vi "3D Scan.vi"() -> ()   [LabVIEW 2011]
uses:
  Global 1.vi
panel:
  in  "Path":path
  in  "Save?":bool
  in  "Stop Button":bool
  out "Position":dbl[](array[numeric]) format="%.6f"
  out "Spectrogram:":dbl[][](graph)
  in  "Update Rate (Hz)":dbl=100000.0
  in  "Y Parameters":T1
  in  "X Parameters":T2
  in  "Scan parameters":T3
  in  "stop 2":bool
  in  "RS232 settings":cluster{"Portnumber":i32, "Baudrate":u16}={"Portnumber"=0, "Baudrate"=4} {"Portnumber" items=["COM1", "COM2", "COM3", "COM4", "COM5", "COM6", "COM7", "COM8", "COM9", "COM10", "COM11", "COM12", "COM13", "COM14", "COM15", "COM16", "COM17", "COM18", "COM19", "COM20", "COM21", "COM22", "COM23", "COM24", "COM25", "COM26", "COM27", "COM28", "COM29", "COM30"]; "Baudrate" items=["9600", "14400", "19200", "38400", "57600", "115200"]}
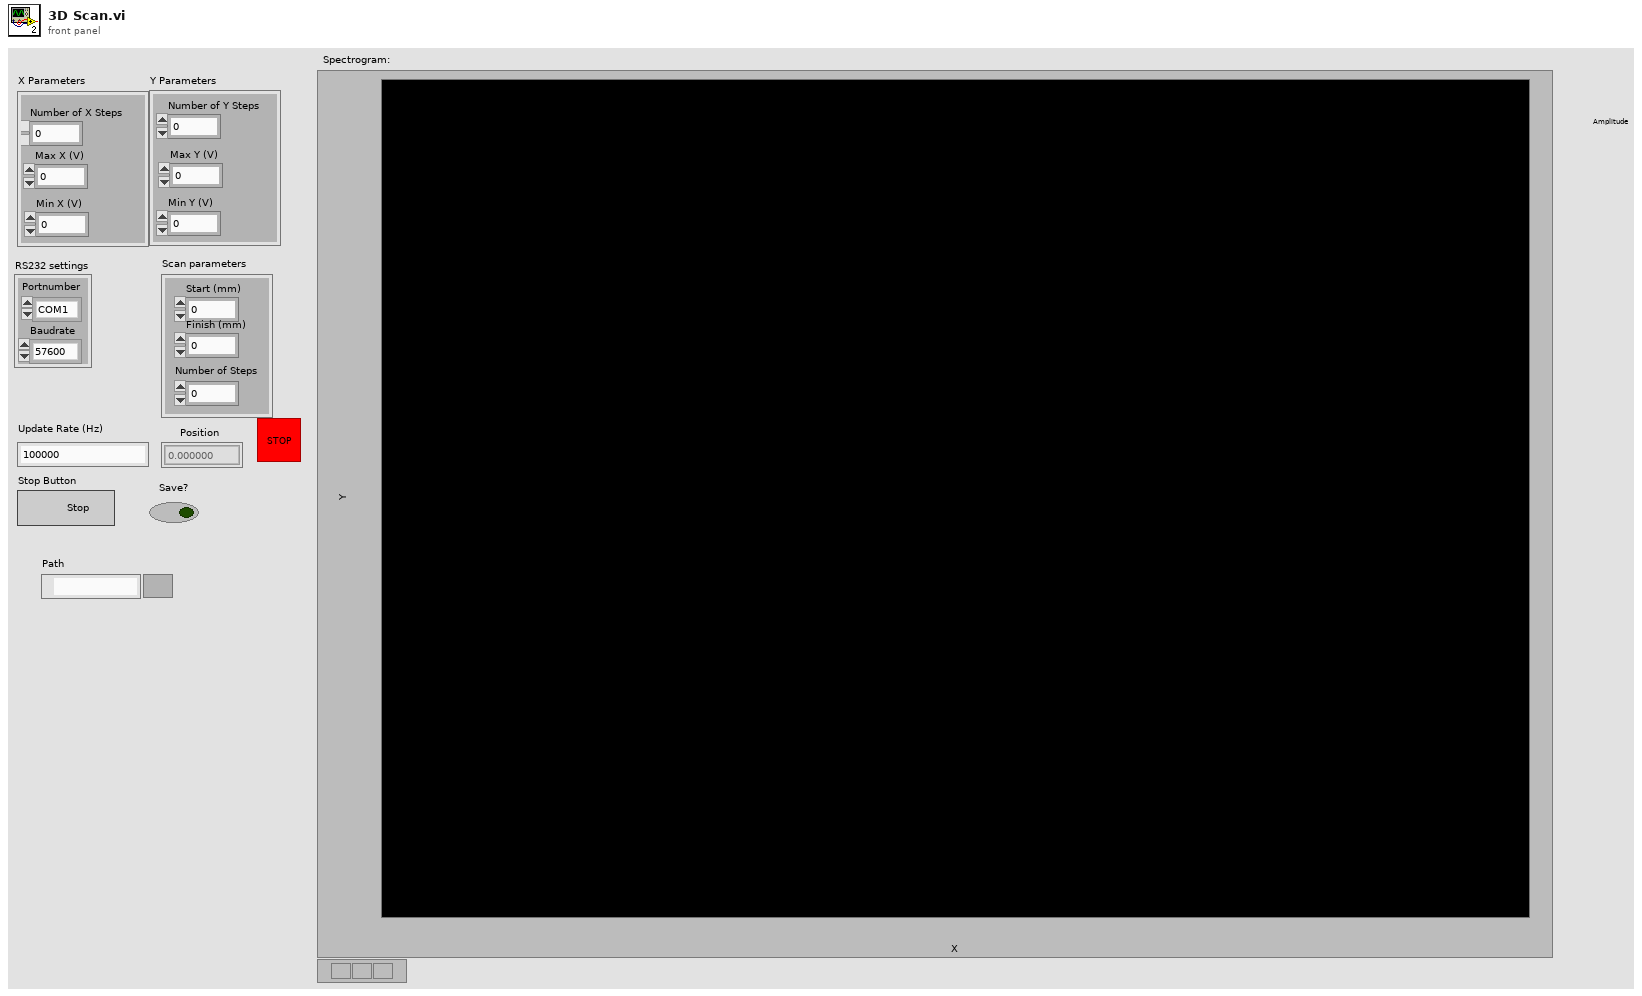
[diagram p1: front panel]
types:
  T1 = cluster{"Number of Y Steps":i32, "Max Y (V)":dbl, "Min Y (V)":dbl}
  T2 = cluster{"Number of X Steps":i32, "Max X (V)":dbl, "Min X (V)":dbl}
  T3 = cluster{"Number of Steps":i32, "Start (mm)":dbl, "Finish (mm)":dbl}
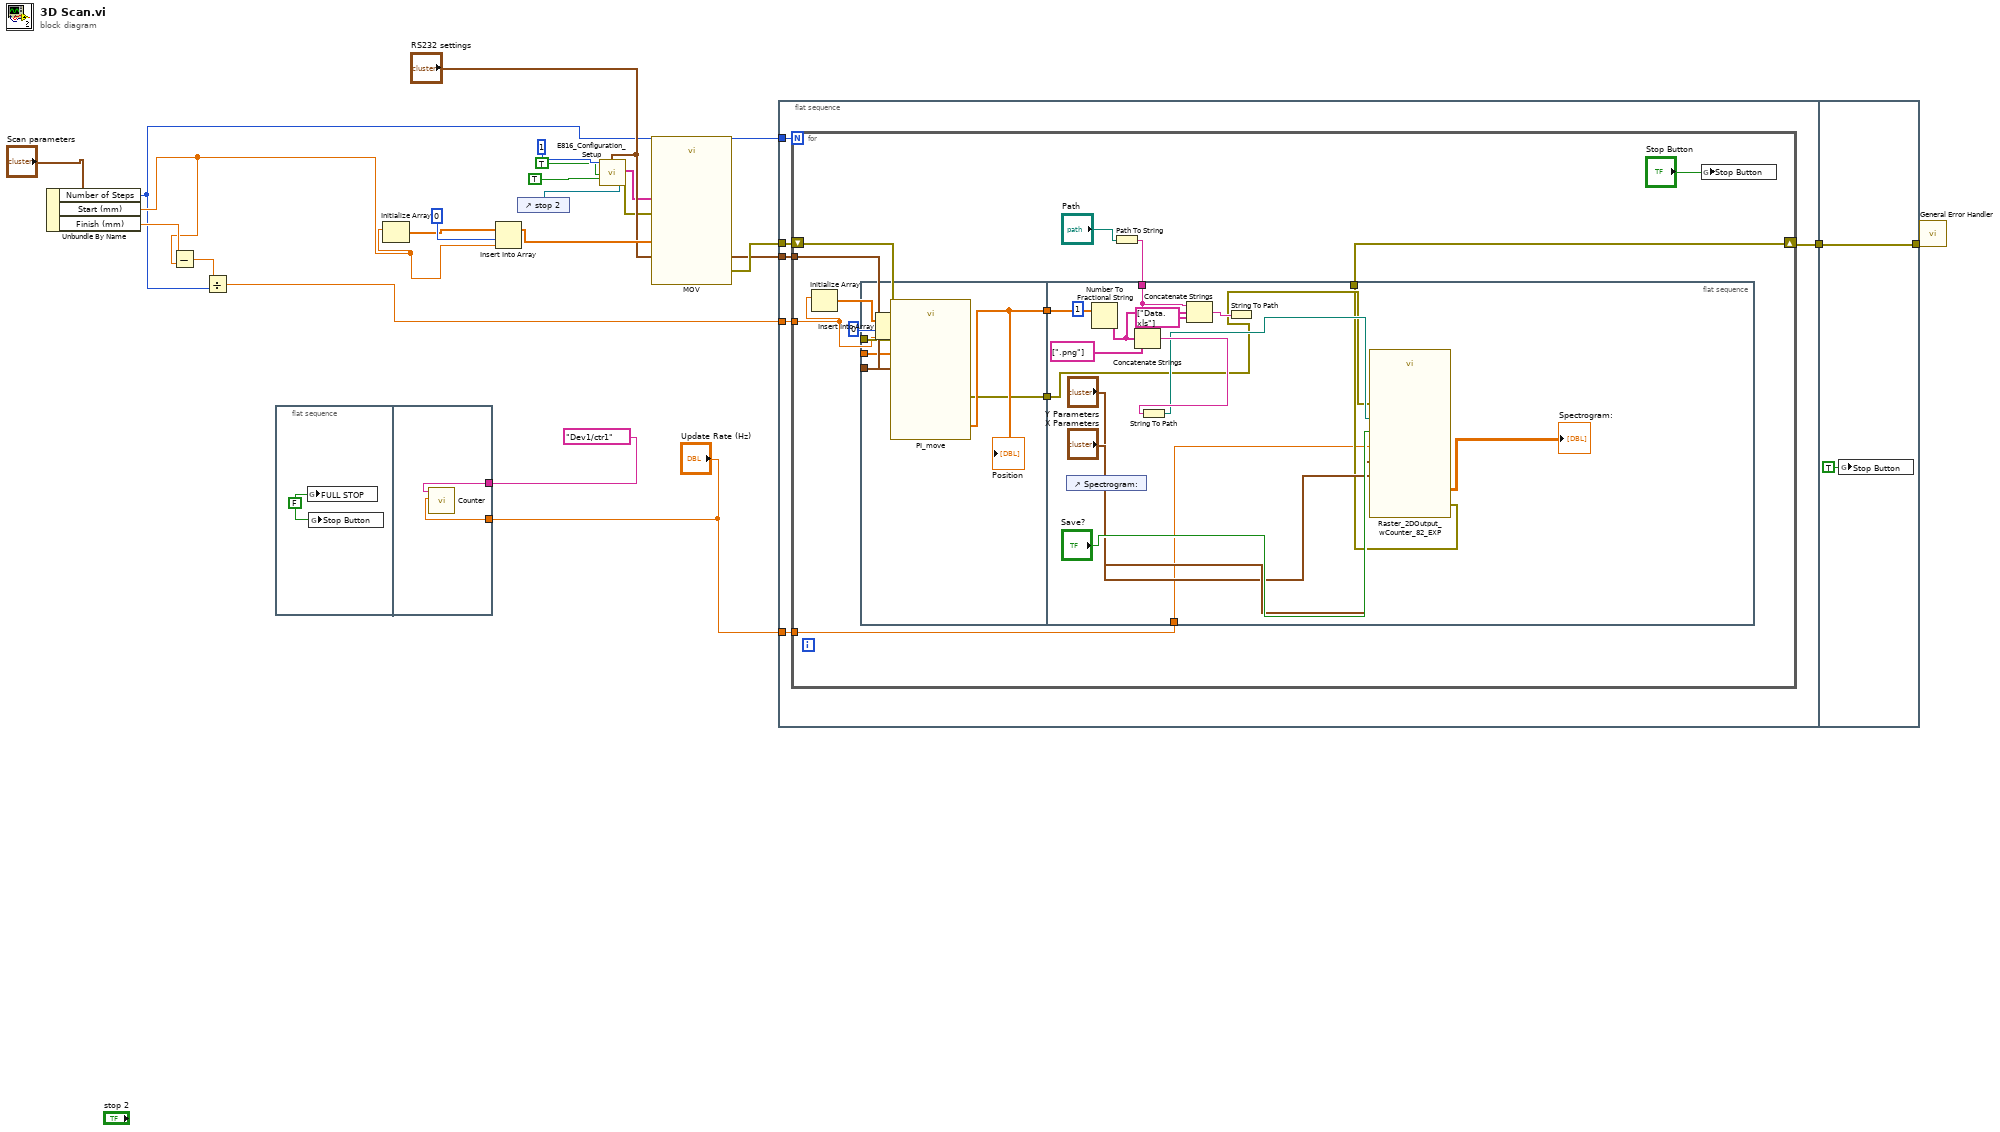
[diagram p0: block diagram]
diagram:
  n1 = Unbundle By Name("Scan parameters") -> ("Number of Steps"=w5:i32, "Start (mm)"=w6:dbl, "Finish (mm)"=w7:dbl)
  n2 = Subtract(x=w7, y=w6) -> (x-y=w21:dbl)
  n3 = Divide(x=w21, y=w5) -> (x/y=w20:dbl)
  n4 = flat-sequence {
    tunnel: tag "Dev1/ctr1" ("Counter(s)") -> [w24]
    tunnel: "Update Rate (Hz)" -> [w23]
    frame #0 {
      w22 = FALSE ("Stop Button")
      n5 = global write "Global 1.vi" "FULL STOP"(w22) -> ()
      n6 = global write "Global 1.vi" "Stop Button"(w22) -> ()
    }
    frame #1 {
      n7 = call "Counter.vi"("Counter(s)"=w24, "Frequency"=w23) -> ()  [unwired: 7 in]
    }
  }
  n8 = Initialize Array(w6) -> (w17:dbl[])  [unwired: 1 in]
  n9 = Insert Into Array(array=w17, index=0, new element=w6) -> (w16:dbl[])
  n10 = control-ref of="stop 2"() -> (w14:refnum<vi>)
  n11 = call "E816_Configuration_Setup.vi"("System no."=1, "All axes?"=TRUE, "Change servo \nstatus to ON?"=TRUE ("Use dialog to define\nconnected stages?"), "RS232 settings"="RS232 settings", "Stop refnum"=w14) -> ("Conn. Axes"=w10:string[], "error out"=w9:errorcluster)  [unwired: 11 in, 2 out]
  n12 = call "MOV.vi"("Axes to move"=w10, "Position values"=w16, "error in"=w9) -> ("error out"=w19:errorcluster)  [unwired: 16 in]
  n13 = flat-sequence {
    tunnel: w20 -> [w30]
    tunnel: w19 -> [w29]
    tunnel: "RS232 settings" -> [w28]
    tunnel: w5 -> [w27]
    tunnel: "Update Rate (Hz)" -> [w25]
    tunnel: [w26] -> w1
    tunnel: [w66] -> w4
    tunnel: w1 -> [w66]
    frame #0 {
      n14 = for {
        N: w27 -> [_]
        tunnel: w28 -> [w43]
        tunnel: w30 -> [w38]
        shift-right: [w31] -> w26
        shift-left: w29 -> [w39]
        tunnel: w25 -> [w34]
        n15 = Initialize Array(w38) -> (w40:dbl[])  [unwired: 1 in]
        n16 = flat-sequence {
          tunnel: w43 -> [w48]
          tunnel: w41 -> [w47]
          tunnel: w39 -> [w46]
          tunnel: [w45] -> w37
          tunnel: [w44] -> w36
          tunnel: w37 -> [w62]
          tunnel: w36 -> [w55]
          tunnel: w34 -> [w49]
          tunnel: w32 -> [w60]
          tunnel: [w50] -> w31
          frame #0 {
            n17 = call "PI_move.vi"("RS232 settings"=w48, "Position values"=w47, "error in"=w46) -> ("Position"=w45:dbl[], "error out"=w44:errorcluster)  [unwired: 14 in, 1 out]
            "Position" <- w45
          }
          frame #1 {
            n18 = control-ref of="Spectrogram:"() -> ()  [unwired: 1 out]
            n19 = Number To Fractional String(number=w62, width (-)=i16 1) -> (F-format string=w59:string[])  [unwired: 2 in]
            n20 = Concatenate Strings(w60, w59, string[] [".png"] ("string")) -> (w64:string)
            n21 = String To Path(string=w64) -> (path=w56:path)
            n22 = Concatenate Strings(w60, w59, string[] ["Data.xls"] ("string")) -> (w57:string)
            n23 = String To Path(string=w57) -> ()  [unwired: 1 out]
            n24 = call "Raster_2DOutput_wCounter_82_EXP.vi"("Save File path"=w56, "Save?"="Save?", "error in"=w55, "Update Rate (Hz)"=w49, "Y Parameters"="Y Parameters", "X Parameters"="X Parameters") -> ("error out"=w50:errorcluster, "Spectrogram:"=→"Spectrogram:":dbl[][])  [unwired: 2 in]
          }
        }
        n25 = Insert Into Array(array=w40, index=0, new element=w38) -> (w41:dbl[])
        n26 = Path To String(path="Path") -> (string=w32:string)
        n27 = global write "Global 1.vi" "Stop Button"("Stop Button") -> ()
      }
    }
    frame #1 {
      n28 = global write "Global 1.vi" "Stop Button"(TRUE ("Stop Button")) -> ()
    }
  }
  n29 = call <vilib>:"General Error Handler.vi"("error in (no error)"=w4) -> ()  [unwired: 10 in, 5 out]
